vi "Pockels-Prevent minimum voltage.vi"(11 "Pockels Value":dbl) -> (1 "Minimum voltage attempt":bool, 2 "Pockels voltage min":dbl format="%#_13g", 3 "Pockels Value (minimum prevented)":dbl)   [LabVIEW 2017]
uses:
  Globals/gl_Pockels control globals.vi
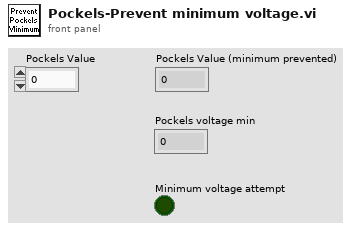
[diagram p1: front panel]
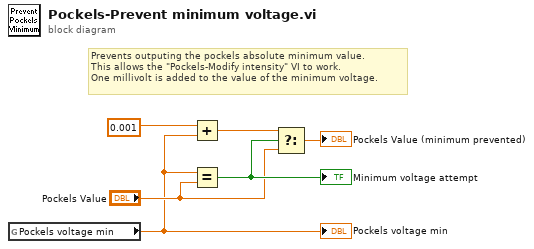
[diagram p0: block diagram]
diagram:
  # "Prevents outputing the pockels absolute minimum value.\nThis allows the \"Pockels-Modify intensity\" VI to work.\nOne millivolt is added to the value of the minimum voltage."
  n1 = global read "gl_Pockels control globals.vi" "Pockels voltage min"() -> (w1:dbl)
  "Pockels voltage min" <- w1
  n2 = Add(x=0.001 ("y"), y=w1) -> (x+y=w4:dbl)
  n3 = Equal?(x=w1, y="Pockels Value") -> (x = y?=w5:bool)
  "Minimum voltage attempt" <- w5
  n4 = Select(t=w4, s=w5, f="Pockels Value") -> (s? t:f=→"Pockels Value (minimum prevented)":dbl)
